vi "Configure Frequency.vi"   [LabVIEW 2013, in "Template - Spectrum Analyzer.lvlib"]
doc: "Configures the frequency range for the spectrum analyzer."
uses:
  <instrlib>/_Template - Spectrum Analyzer/Template - Spectrum Analyzer.lvlib
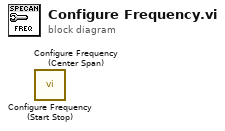
[diagram p0: block diagram]
diagram:
  n1 = call <instrlib>:"Configure Frequency (Start Stop).vi"() -> ()  [unwired: 10 in, 2 out]
  n2 = call <instrlib>:"Configure Frequency (Center Span).vi"() -> ()  [unwired: 10 in, 2 out]
